vi "Strings to Slave Configuration.vi"(10 "Filter":string[][](array[string]), 11 "Gas":string[][](array[string])) -> (2 "Filter Sequences Out":T1[](array[typedef]), 3 "Gas Mixtures Out":T2[](array[typedef]) {"ADC Gains" items=["0"=0, "3"=3, "4"=4, "5"=5, "6"=6, "7"=7]})   [LabVIEW 2015]
uses:
  Tests/Controls/Gas Mixture.ctl
  CAN Communication/PAS/Typedefs/ADC Gains.ctl
  Tests/Controls/Filter Sequence.ctl
  CAN Communication/PAS/PAS.lvclass
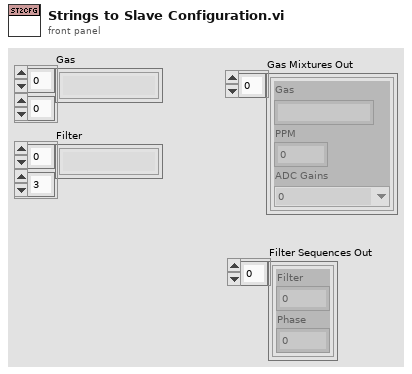
[diagram p1: front panel]
types:
  T1 = typedef "Filter Sequence.ctl" = cluster{"Filter":u8, "Phase":dbl}
  T2 = typedef "Gas Mixture.ctl" = cluster{"Gas":string, "PPM":dbl, "ADC Gains":T3}
  T3 = typedef "PAS.lvclass/ADC Gains.ctl" = u16
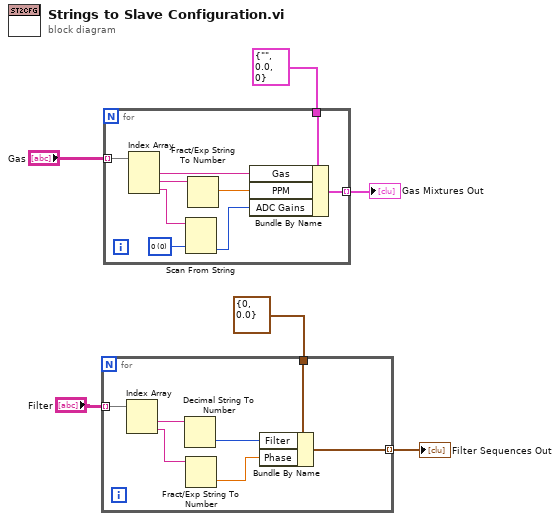
[diagram p0: block diagram]
diagram:
  n1 = for {
    tunnel: "Filter" -> [w13] mode=indexing
    tunnel: T1 {"Filter"=0, "Phase"=0.0} ("Filter Sequence") -> [w12]
    tunnel: [w7] -> w1 mode=indexing
    n2 = Index Array(array=w13) -> (element #1=w11:string, element #2=w9:string)  [unwired: 2 in]
    n3 = Decimal String To Number(string=w11) -> (number=w10:i32)  [unwired: 2 in, 1 out]
    n4 = Fract/Exp String To Number(string=w9) -> (number=w8:dbl)  [unwired: 3 in, 1 out]
    n5 = Bundle By Name(cluster=w12, "Filter"=w10, "Phase"=w8) -> (w7:T1)
  }
  "Filter Sequences Out" <- w1
  n6 = for {
    tunnel: "Gas" -> [w22] mode=indexing
    tunnel: T2 {"Gas"="", "PPM"=0.0, "ADC Gains"=0} ("Gas Mixture") -> [w18]
    tunnel: [w14] -> w4 mode=indexing
    w16 = T3 0 items=["0"=0, "3"=3, "4"=4, "5"=5, "6"=6, "7"=7] ("ADC Gains")
    n7 = Index Array(array=w22) -> (element #1=w21:string, element #2=w20:string, element #3=w17:string)  [unwired: 3 in]
    n8 = Scan From String(input string=w17, default 1=w16) -> (output 1=w15:T3)  [unwired: 3 in, 3 out]
    n9 = Fract/Exp String To Number(string=w20) -> (number=w19:dbl)  [unwired: 3 in, 1 out]
    n10 = Bundle By Name(cluster=w18, "Gas"=w21, "PPM"=w19, "ADC Gains"=w15) -> (w14:T2)
  }
  "Gas Mixtures Out" <- w4
